vi "get channel features.vi"(8 "error in (no error)":errorcluster, 11 "channel handle":u16 format="%x") -> (0 "error out":errorcluster, 3 "features":T1)   [LabVIEW 2024, in "atsj peakcan basic.lvlib"]
uses:
  atsj peakcan basic.lvlib
  parameter.ctl
  get parameter - i32.vi
  features.ctl
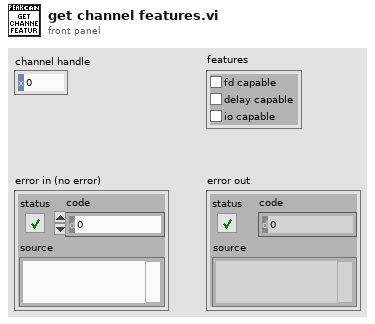
[diagram p1: front panel]
types:
  T1 = typedef "atsj peakcan basic.lvlib/features.ctl" = cluster{"fd capable":bool, "delay capable":bool, "io capable":bool}
  T2 = typedef "atsj peakcan basic.lvlib/parameter.ctl" = enum8{"DEVICE_ID", "5VOLTS_POWER", "RECEIVE_EVENT", "MESSAGE_FILTER", "API_VERSION", "CHANNEL_VERSION", "BUSOFF_AUTORESET", "LISTEN_ONLY", "LOG_LOCATION", "LOG_STATUS", "LOG_CONFIGURE", "LOG_TEXT", "CHANNEL_CONDITION", "HARDWARE_NAME", "RECEIVE_STATUS", "CONTROLLER_NUMBER", "TRACE_LOCATION", "TRACE_STATUS", "TRACE_SIZE", "TRACE_CONFIGURE", "CHANNEL_IDENTIFYING", "CHANNEL_FEATURES", "BITRATE_ADAPTING", "BITRATE_INFO", "BITRATE_INFO_FD", "BUSSPEED_NOMINAL", "BUSSPEED_DATA", "IP_ADDRESS", "LAN_SERVICE_STATUS", "ALLOW_STATUS_FRAMES", "ALLOW_RTR_FRAMES", "ALLOW_ERROR_FRAMES", "INTERFRAME_DELAY", "ACCEPTANCE_FILTER_11BIT", "ACCEPTANCE_FILTER_29BIT", "IO_DIGITAL_CONFIGURATION", "IO_DIGITAL_VALUE", "IO_DIGITAL_SET", "IO_DIGITAL_CLEAR", "IO_ANALOG_VALUE", "FIRMWARE_VERSION", "ATTACHED_CHANNELS_COUNT", "ATTACHED_CHANNELS", "ALLOW_ECHO_FRAMES", "DEVICE_PART_NUMBER", "HARD_RESET_STATUS", "LAN_CHANNEL_DIRECTION", "DEVICE_GUID"}
  T3 = cluster{"Boolean array[0]":bool, "Boolean array[1]":bool, "Boolean array[2]":bool}
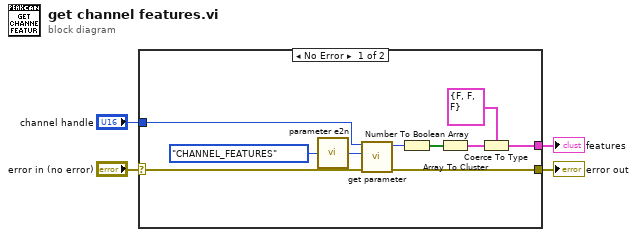
[diagram p0: block diagram]
diagram:
  n1 = case shown="No Error" "error in (no error)" {
    selector: "error in (no error)" -> [w12 w15]
    tunnel: [w11 w15] -> w3
    tunnel: "channel handle" -> [w10 _]
    tunnel: [w5 _] -> w1
    frame No Error {
      n2 = call "parameter e2n.vi"("parameter"=parameter."CHANNEL_FEATURES") -> ("number"=w13:u8)
      n3 = call-poly "get parameter.vi"("error in (no error)"=w12, "parameter"=w13, "channel"=w10) -> ("error out"=w11:errorcluster, "value"=w9:i32)  [unwired: 7 in]
      n4 = Number To Boolean Array(number=w9) -> (Boolean array=w8:bool[])
      n5 = Array To Cluster(array=w8) -> (cluster=w7:T3)
      n6 = Coerce To Type(0:w7, 1:T1 {"fd capable"=FALSE, "delay capable"=FALSE, "io capable"=FALSE}) -> (2:w5:T1)
    }
    frame Error {
    }
  }
  "error out" <- w3
  "features" <- w1
